vi "CastToMoreGenericClass.vi"(11 "Sequence Context In":refnum<k7>) -> (0 "error out":errorcluster, 2 "Comment":string, 3 "Version":string)   [LabVIEW 2011]
doc: "This VI demonstrates how to cast a SequenceFile object in order access properties of the PropertyObjectFile and PropertyObject parent classes."
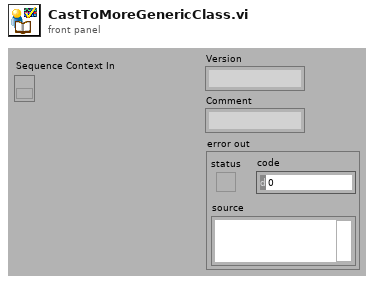
[diagram p1: front panel]
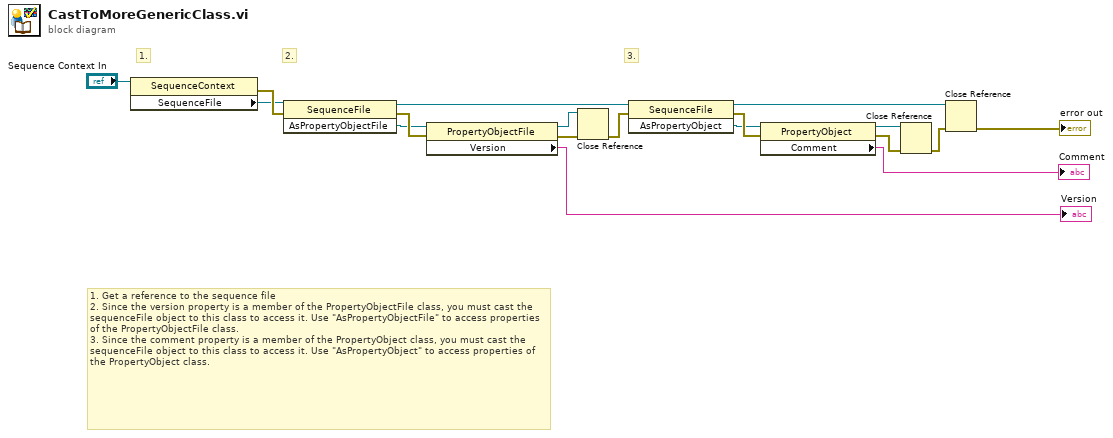
[diagram p0: block diagram]
diagram:
  # "1. Get a reference to the sequence file\n2. Since the version property is a member of the PropertyObjectFile class, you must cast the sequenceFile object to this class to access it. Use \"AsPropertyObjectFile\" to access properties of the PropertyObjectFile class.\n3. Since the comment property is a member of the PropertyObject class, you must cast the sequenceFile object to this class to access it. Use \"AsPropertyObject\" to access properties of the PropertyObject class."
  # "3."
  # "2."
  # "1."
  n1 = property class="SequenceContext"(reference="Sequence Context In") -> (error out=w17:errorcluster, "SequenceFile"=w6:refnum<k7>)  [unwired: 1 in, 1 out]
  n2 = invoke class="SequenceFile" method="AsPropertyObjectFile"(reference=w6, error in=w17) -> (reference out=w3:refnum<k7>, error out=w16:errorcluster, "AsPropertyObjectFile"=w11:refnum<k7>)  [unwired: 1 in]
  n3 = property class="PropertyObjectFile"(reference=w11, error in=w16) -> (reference out=w8:refnum<k7>, error out=w9:errorcluster, "Version"=→"Version":string)
  n4 = Close Reference(reference=w8, error in (no error)=w9) -> (error out=w2:errorcluster)
  n5 = invoke class="SequenceFile" method="AsPropertyObject"(reference=w3, error in=w2) -> (reference out=w10:refnum<k7>, error out=w15:errorcluster, "AsPropertyObject"=w14:refnum<k7>)  [unwired: 1 in]
  n6 = property class="PropertyObject"(reference=w14, error in=w15) -> (reference out=w13:refnum<k7>, error out=w12:errorcluster, "Comment"=→"Comment":string)
  n7 = Close Reference(reference=w13, error in (no error)=w12) -> (error out=w4:errorcluster)
  n8 = Close Reference(reference=w10, error in (no error)=w4) -> (error out=→"error out":errorcluster)
